vi "CreateWidget.vi"(6 "control name":string, 7 "PythonConverter_GUI in":refnum<class "PythonConverter_GUI.lvclass">, 8 "error in":errorcluster, 11 "Control in":refnum<class "Control.lvclass">) -> (0 "error out":errorcluster, 1 "get image":bool, 2 "module":T1, 3 "Control out":refnum<class "Control.lvclass">, 4 "control":string, 5 "PythonConverter_GUI out":refnum<class "PythonConverter_GUI.lvclass">)   [LabVIEW 2014, in "PythonConverter_GUI.lvclass"]
uses:
  PythonConverter_GUI.lvclass
  VI Interpreter/Classes/Control/Control.lvclass
  TypeDefs/PythonModuleTD.ctl
  Parsing/Python Functions.lvlib
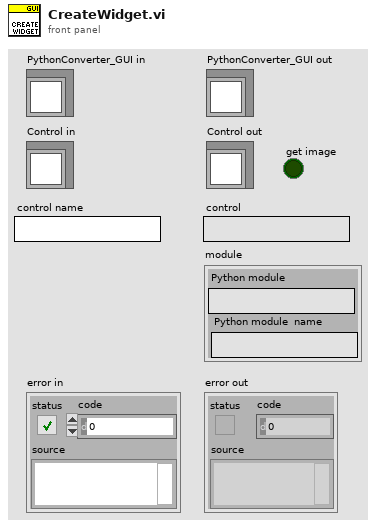
[diagram p1: front panel]
types:
  T1 = typedef "PythonConverter_GUI.lvclass/PythonModuleTD.ctl" = cluster{"Python module":string, "Python module  name":string}
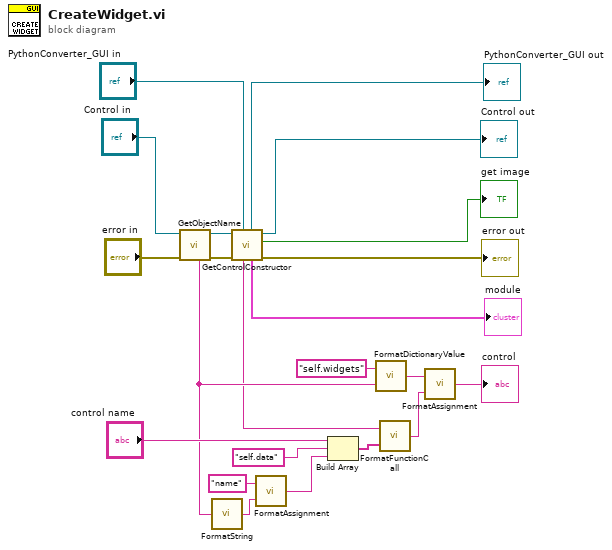
[diagram p0: block diagram]
diagram:
  n1 = call-dynamic "GetObjectName.vi"("error in"="error in", "GObject in"="Control in") -> ("error out"=w8:errorcluster, "GObject out"=w9:refnum<class "Control.lvclass">, "Name"=w10:string)  [unwired: 5 in]
  n2 = call "FormatString.vi"("value"=w10) -> ("python object"=w16:string)
  n3 = call "GetControlConstructor.vi"("PythonConverter_GUI in"="PythonConverter_GUI in", "error in"=w8, "Control in"=w9) -> ("error out"=→"error out":errorcluster, "get image"=→"get image":bool, "Control out"=→"Control out":refnum<class "Control.lvclass">, "module"=→"module":T1, "PythonConverter_GUI out"=→"PythonConverter_GUI out":refnum<class "PythonConverter_GUI.lvclass">, "constructor"=w4:string)  [unwired: 3 in]
  n4 = call "FormatAssignment.vi"("value"=w16, "name"="name") -> ("python assignment"=w14:string)
  n5 = Build Array("control name", "self.data" ("String"), w14) -> (w17:string[])
  n6 = call "FormatDictionaryValue.vi"("key"=w10, "dictionary"="self.widgets") -> ("python object"=w19:string)
  n7 = call "FormatFunctionCall.vi"("parameters"=w17, "function"=w4) -> ("python object"=w18:string)
  n8 = call "FormatAssignment.vi"("value"=w18, "name"=w19) -> ("python assignment"=→"control":string)
